vi "DAB_Cosimulation.vi"() -> ()   [LabVIEW 2017]
uses:
  <vilib>/rvi/Analysis/control/PID/Typedef/niFpgaPID_PIGains.ctl
  <vilib>/Simulation/Scripting/Companion Diagram/SimConfigNode/SimParams.ctl
  <vilib>/Simulation/Scripting/Companion Diagram/SimConfigNode/_simSolvers.ctl
  <vilib>/Simulation/Implementation/Shared/SIMSCR Execution Mode.ctl
  <vilib>/rvi/Analysis/control/PID/Typedef/niFpgaPID_OutputRange.ctl
  <vilib>/Simulation/Param Hierarchy/Typedefs/SIMPH Param Control Actions.ctl
  <vilib>/rvi/Analysis/control/PID/Typedef/niFpgaPID_PIErrors.ctl
  <vilib>/rvi/Analysis/control/PID/Typedef/niFpgaPID_PIState.ctl
  <vilib>/Simulation/Implementation/Shared/NILVSim_ParamChanged.vi
  <vilib>/Simulation/Implementation/Shared/NILVSIM_BeginStep.vi
  <vilib>/Simulation/Utility/Implementation/SIM Halt.vi
  <vilib>/Simulation/Implementation/Shared/NILVSim_Manager.vi
  <vilib>/Utility/error.llb/Clear Errors.vi
  <vilib>/Simulation/Implementation/Shared/NILVSim_FinalizeModel.vi
  <vilib>/Simulation/Implementation/Shared/SIM Unbundle Sim Info.vi
  <vilib>/Simulation/Implementation/Shared/NILVSim_Initialize.vi
  PhaseShiftModulation.vi
  <vilib>/Simulation/Utility/Implementation/NILVSim Get Time and IsAcceptedStep.vi
  <vilib>/Simulation/Implementation/Shared/SIMSH Read Queue.vi
  <vilib>/Simulation/Implementation/Shared/NILVSim_GetModelError.vi
  <vilib>/Simulation/Implementation/Shared/SIM Bundle Sim Info.vi
  <vilib>/Simulation/Scripting/Companion Diagram/SimConfigNode/SimDog.xnode
  <vilib>/Simulation/Implementation/XNodeFramework/SimXNode/SimX.xnode
  <vilib>/Simulation/EMI/Plugins/Multisim Design/MultisimEMICtrl.dll
  <vilib>/Simulation/Implementation/Shared/NI_SIM_Implementation.lvlib
panel:
  out "Batt_Current":dbl=12.354476241061633
  out "Battery Voltage":dbl=24.24708923819107
  out "Xfmr Current":dbl=5.961545821791743
  out "Power":dbl=299.5600879081328
  in  "Halt?":bool
  out "DAB_Currents":dbl[][](graph)=[[5.961545821791743, 24.24708923819107, 12.354476241061633]]
  in  "gains":T1={"proportional gain"=10.0, "integral gain"=0.005} {"proportional gain" step=0.125}
  in  "Power_Setpoint":dbl=300.0 format="%#_13g"
  out "DAB_Power":dbl(graph)=299.5600879081328
  in  "enable":bool=TRUE
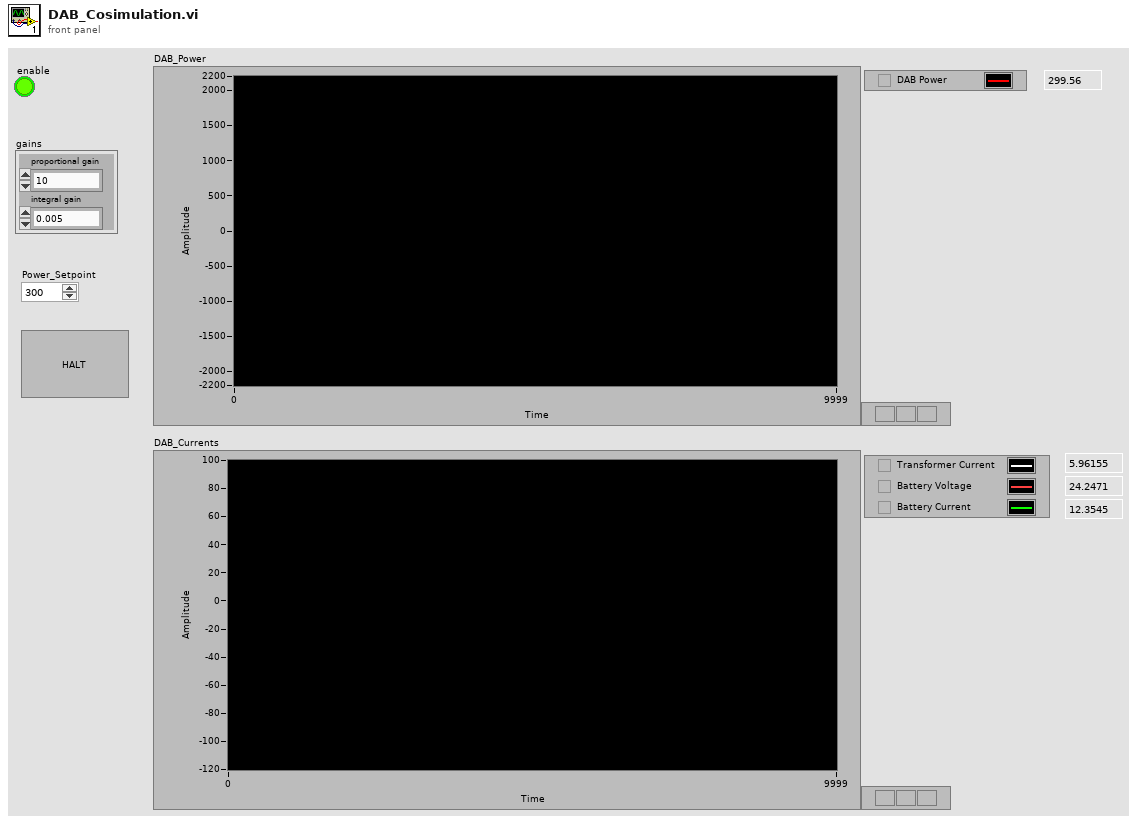
[diagram p1: front panel]
types:
  T1 = typedef "niFpgaPID_PIGains.ctl" = cluster{"proportional gain":sgl, "integral gain":sgl}
  T2 = typedef "niFpgaPID_OutputRange.ctl" = cluster{"output high (Inf)":sgl, "output low (-Inf)":sgl}
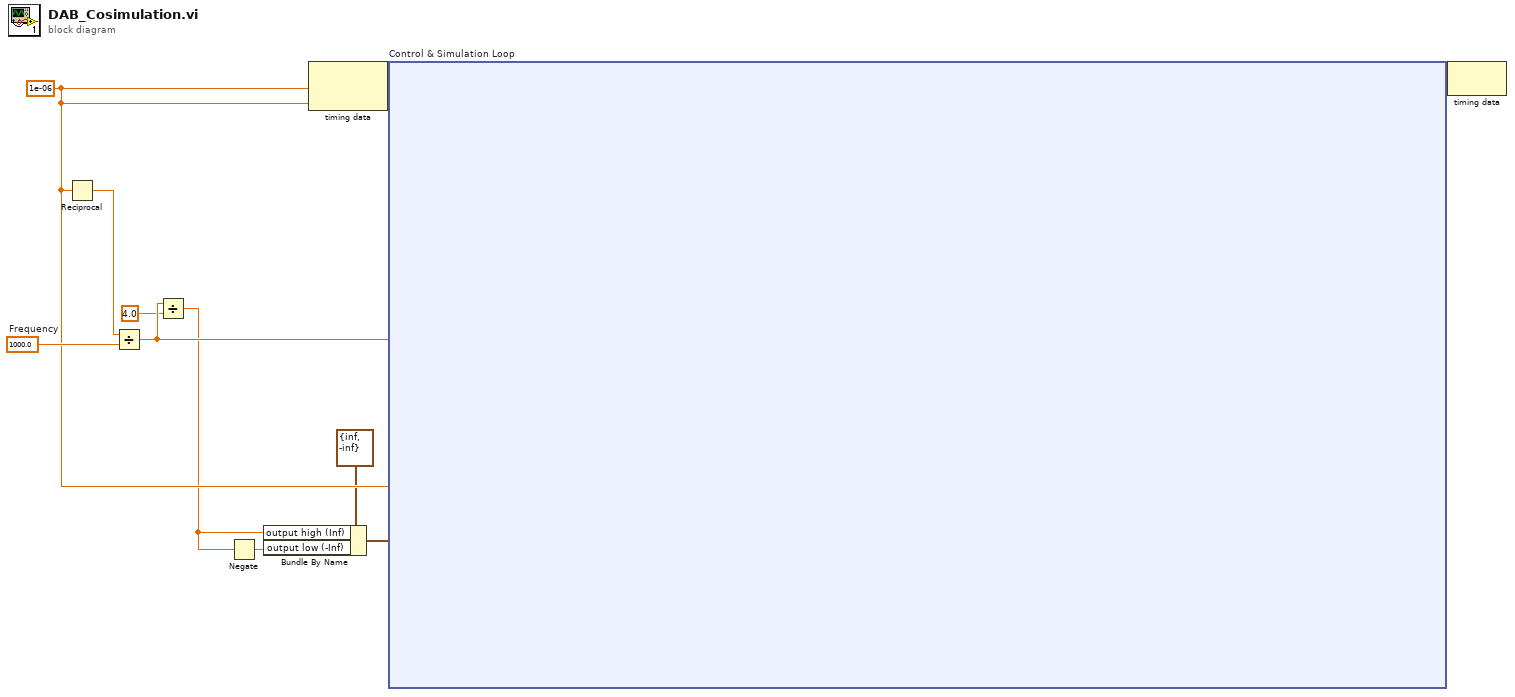
[diagram p0: block diagram]
diagram:
  w9 = 1000.0  # Frequency
  w3 = 1e-06 ("Step Size (s)")
  n1 = Reciprocal(x=w3) -> (1/x=w8:dbl)
  n2 = Divide(x=w8, y=w9) -> (x/y=w7:dbl)
  n3 = Divide(x=w7, y=4.0) -> (x/y=w1:dbl)
  n4 = Negate(x=w1) -> (-x=w5:dbl)
  n5 = Bundle By Name(cluster=T2 {"output high (Inf)"=inf, "output low (-Inf)"=-inf} ("output range"), "output high (Inf)"=w1, "output low (-Inf)"=w5) -> (w4:T2)
  n6 = node-c288(w3, w3) -> (w11:variant)
  n7 = node-c254 "Control & Simulation Loop"(w11, w7, w4, w3) -> (w10:variant)
  n8 = node-c288(w10) -> ()  [unwired: 1 out]
